vi "불리언연산.vi"() -> ()   [LabVIEW 2014]
panel:
  out "D":bool=TRUE
  in  "C":bool
  in  "B":bool
  in  "A":bool=TRUE
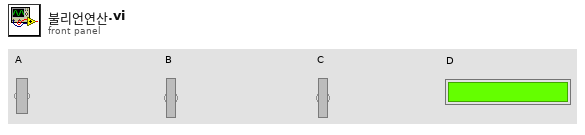
[diagram p1: front panel]
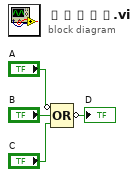
[diagram p0: block diagram]
diagram:
  n1 = Compound Arithmetic op=OR(invert "A", "B", "C") -> (invert →"D":bool)
